vi "FilterNonAlphaNumeric.vi"(4 "String In":string) -> (1 "String out":string)   [LabVIEW 2022 SP3]
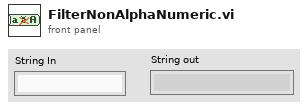
[diagram p1: front panel]
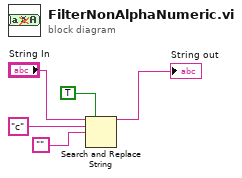
[diagram p0: block diagram]
diagram:
  n1 = Search and Replace String(replace all?=TRUE ("replace all? (F)"), input string="String In", search string="c", replace string="") -> (result string=→"String out":string)  [unwired: 4 in, 3 out]
